vi "Get Label data.vi"(8 "error in (no error)":errorcluster, 11 "Variant":string) -> (0 "error out":errorcluster, 1 "Variant not found":bool, 2 "HardwareVersion":string, 3 "SoftwareVersion":string)   [LabVIEW 2023]
uses:
  <vilib>/Utility/config.llb/Read Key (String).vi
  <vilib>/Utility/config.llb/NI_LVConfig.lvlib
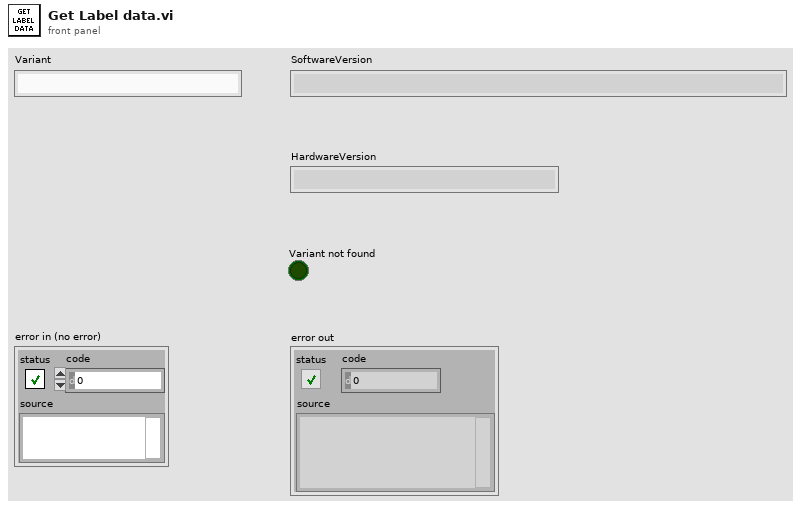
[diagram p1: front panel]
types:
  T1 = typedef "NI_LVConfig.lvlib/Config Data RefNum.ctl" = refnum<k1>
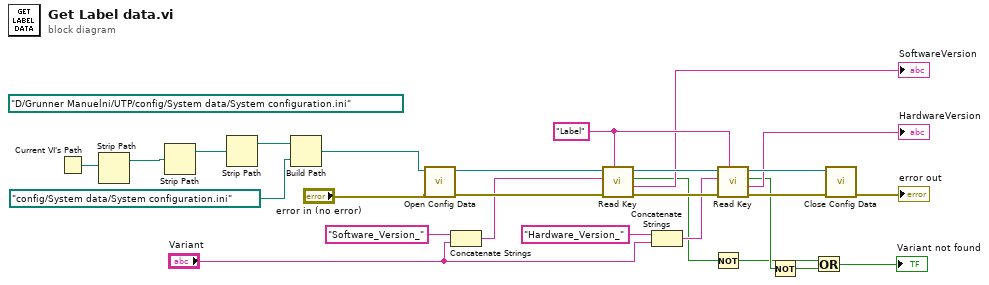
[diagram p0: block diagram]
diagram:
  w14 = "Label" ("section")
  (unwired) path "D:/Grunner Manuelni/UTP/config/System data/System configuration.ini" ("configuration file path")
  n1 = Current VI's Path() -> (path=w3:path)
  n2 = Strip Path(path=w3) -> (stripped path=w2:path)  [unwired: 1 out]
  n3 = Strip Path(path=w2) -> (stripped path=w6:path)  [unwired: 1 out]
  n4 = Strip Path(path=w6) -> (stripped path=w5:path)  [unwired: 1 out]
  n5 = Build Path(base path=w5, name or relative path=path "config/System data/System configuration.ini") -> (appended path=w1:path)
  n6 = call <vilib>:"Open Config Data.vi"("error in (no error)"="error in (no error)", "configuration file path"=w1) -> ("error out"=w25:errorcluster, "refnum"=w24:T1)  [unwired: 7 in, 1 out]
  n7 = Concatenate Strings("Software_Version_" ("key"), "Variant") -> (w18:string)
  n8 = call-poly <vilib>:"Read Key.vi"("section"=w14, "error in (no error)"=w25, "key"=w18, "refnum"=w24) -> ("error out"=w21:errorcluster, "value"=→"SoftwareVersion":string, "found?"=w11:bool, "refnum out"=w23:T1)  [unwired: 4 in]
  n9 = Concatenate Strings("Hardware_Version_" ("key"), "Variant") -> (w15:string)
  n10 = Not(x=w11) -> (.not. x?=w8:bool)
  n11 = call-poly <vilib>:"Read Key.vi"("section"=w14, "error in (no error)"=w21, "key"=w15, "refnum"=w23) -> ("error out"=w20:errorcluster, "value"=→"HardwareVersion":string, "found?"=w10:bool, "refnum out"=w22:T1)  [unwired: 4 in]
  n12 = Not(x=w10) -> (.not. x?=w9:bool)
  n13 = Or(x=w8, y=w9) -> (x .or. y?=→"Variant not found":bool)
  n14 = call <vilib>:"Close Config Data.vi"("error in (no error)"=w20, "refnum"=w22) -> ("error out"=→"error out":errorcluster)  [unwired: 8 in, 1 out]
